vi "RichToFlatpumploop_GetSensorResult.vi"(5 "OutputClusterType":T1, 11 "InputCluster":T3) -> (3 "OutputCluster":T1)   [LabVIEW 2024, in "pumploop_client.lvlib"]
uses:
  pumploop_client.lvlib
  pumploop_GetSensorResult.ctl
  pumploop_Sensors.ctl
  pumploop_GetSensorResult_Flat.ctl
  pumploop_Sensors_Flat.ctl
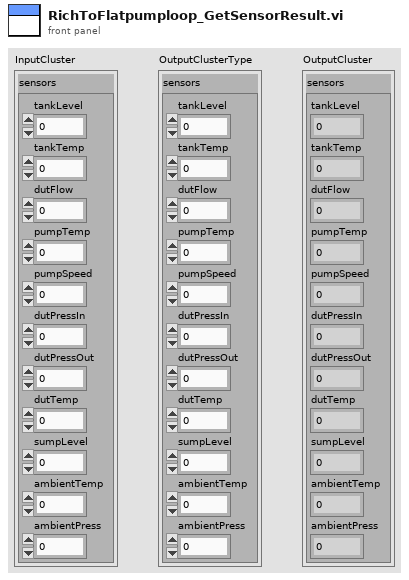
[diagram p1: front panel]
types:
  T1 = typedef "pumploop_client.lvlib/pumploop_GetSensorResult_Flat.ctl" = cluster{"sensors":T2}
  T2 = typedef "pumploop_client.lvlib/pumploop_Sensors_Flat.ctl" = cluster{"tankLevel":sgl, "tankTemp":sgl, "dutFlow":sgl, "pumpTemp":sgl, "pumpSpeed":sgl, "dutPressIn":sgl, "dutPressOut":sgl, "dutTemp":sgl, "sumpLevel":sgl, "ambientTemp":sgl, "ambientPress":sgl}
  T3 = typedef "pumploop_client.lvlib/pumploop_GetSensorResult.ctl" = cluster{"sensors":T4}
  T4 = typedef "pumploop_client.lvlib/pumploop_Sensors.ctl" = cluster{"tankLevel":sgl, "tankTemp":sgl, "dutFlow":sgl, "pumpTemp":sgl, "pumpSpeed":sgl, "dutPressIn":sgl, "dutPressOut":sgl, "dutTemp":sgl, "sumpLevel":sgl, "ambientTemp":sgl, "ambientPress":sgl}
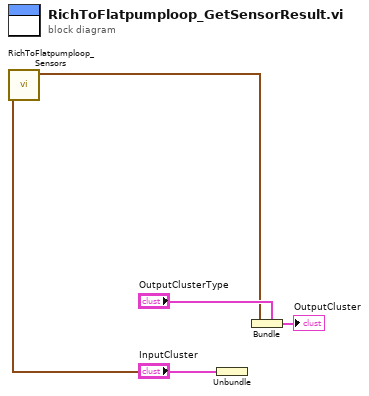
[diagram p0: block diagram]
diagram:
  n1 = Unbundle "Unbundle"("InputCluster") -> ("sensors"=w2:T4)
  n2 = call "RichToFlatpumploop_Sensors.vi"("InputCluster"=w2) -> ("OutputCluster"=w1:T2)  [unwired: 10 in]
  n3 = Bundle "Bundle"(cluster="OutputClusterType", "sensors"=w1) -> (→"OutputCluster":T1)
